vi "Read status mMc.vi"(1 "Port":T1={"P type"=0, "reference"="", " Terminator "="\r\n", "Timeout"=300} {"Timeout" step=10; "P type" items=["none", "RS-232C"]}, 3 "error in (no error)":errorcluster, 5 "Controller #":string) -> (6 "Moving?":bool, 7 "In position?":bool, 9 "error out":errorcluster)   [LabVIEW 2013]
panel:
  out "Error?":bool
  out "status array":bool[](array[boolean])
  # "Read status"
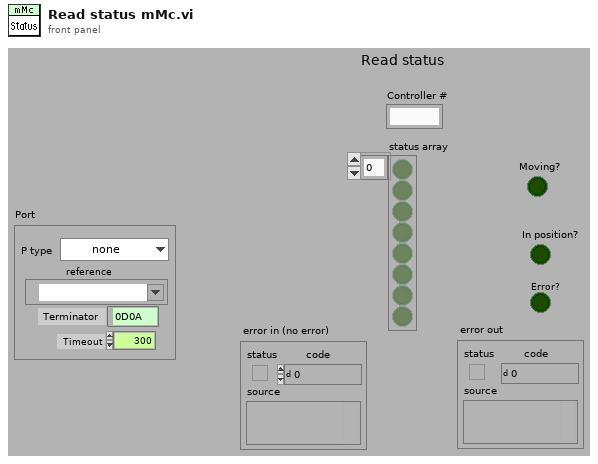
[diagram p1: front panel]
types:
  T1 = cluster{"P type":u16, "reference":refnum<visa-resource-name>, " Terminator ":string, "Timeout":i32}
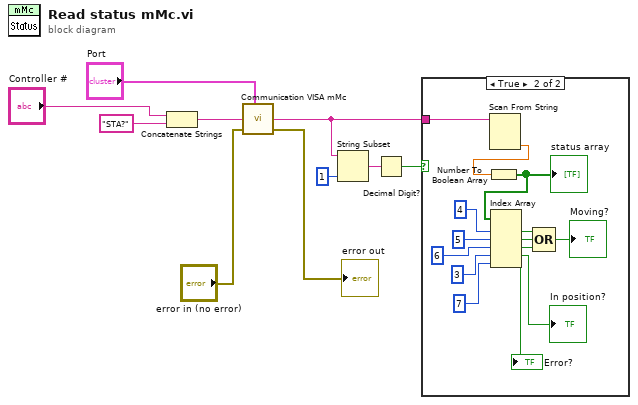
[diagram p0: block diagram]
diagram:
  n1 = Concatenate Strings("Controller #", "STA?") -> (w6:string)
  n2 = call "Communication VISA mMc.vi"("Port"="Port", "Command"=w6, "error in (no error)"="error in (no error)") -> ("Return"=w1:string, "error out"=→"error out":errorcluster)  [unwired: 3 in, 2 out]
  n3 = String Subset(string=w1, length (rest)=1 ("length (rest)")) -> (substring=w3:string)  [unwired: 1 in]
  n4 = Decimal Digit?(1:w3) -> (0:w2:bool)
  n5 = case shown="True" w2 {
    tunnel: w1 -> [_ w24]
    frame False {
    }
    frame True {
      n6 = Scan From String(input string=w24) -> (output 1=w23:dbl)  [unwired: 4 in, 3 out]
      n7 = Number To Boolean Array(number=w23) -> (Boolean array=w22:bool[])
      "status array" <- w22
      n8 = Index Array(array=w22, index #1=4 ("index"), index #2=5 ("index"), index #3=6 ("index"), index #4=3 ("index"), index #5=7 ("index")) -> (element #1=w19:bool, element #2=w18:bool, element #3=w17:bool, element #4=→"In position?":bool, element #5=→"Error?":bool)
      n9 = Compound Arithmetic op=OR(w19, w18, w17) -> (→"Moving?":bool)
    }
  }
